vi "DAC Run.vi"(8 "error in":errorcluster, 11 "DAC HS Vib in":refnum<class "DAC HS Vib.lvclass">) -> (0 "error out":errorcluster, 3 "DAC HS Vib out":refnum<class "DAC HS Vib.lvclass">)   [LabVIEW 2019, in "DAC.lvlib" / "DAC HS Vib.lvclass"]
uses:
  DAC HS Vib.lvclass
  C:/Users/krio/Documents/LV_Projects/test-stand/App/DAC/DAC.lvclass
  DAC.lvclass/DAC.ctl
  Results/Results Method.ctl
  Results/DeepU Results/DeepU Results.lvclass
  DAC HS Vib.lvclass/DAC HS Vib.ctl
  <vilib>/DAQmx/read.llb/DAQmx Read (Analog 1D Wfm NChan NSamp).vi
  <vilib>/DAQmx/miscellaneous.llb/DAQmx Fill In Error Info.vi
  DAC.lvclass
  Results/Results.lvlib
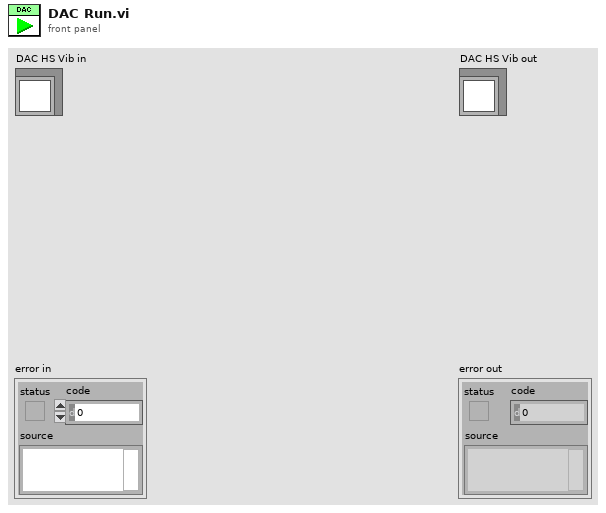
[diagram p1: front panel]
types:
  T1 = typedef "Results.lvlib/Results Method.ctl" = enum16{"Get", "Set"}
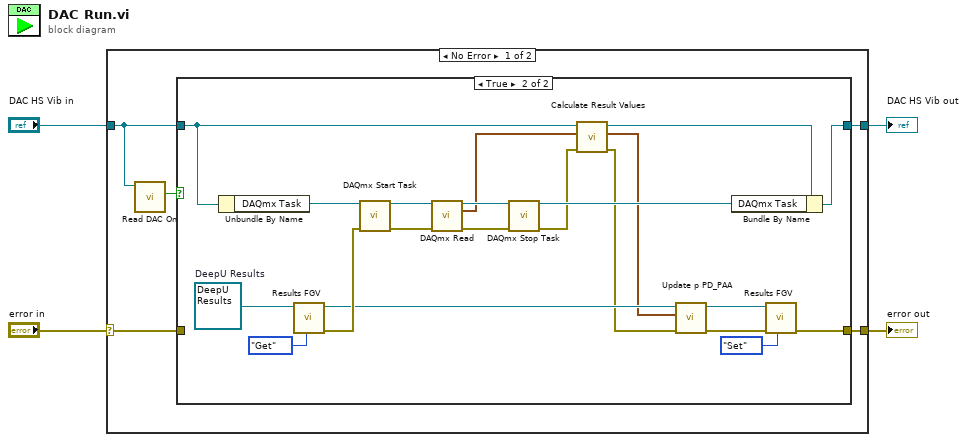
[diagram p0: block diagram]
diagram:
  n1 = case shown="No Error" "error in" {
    selector: "error in" -> [w7 w34]
    tunnel: [w6 w34] -> w2
    tunnel: [w8 w33] -> w1
    tunnel: "DAC HS Vib in" -> [w5 w33]
    frame No Error {
      n2 = call "Read DAC On.vi"("DAC in"=w5) -> ("DAC On"=w9:bool)  [unwired: 8 in, 2 out]
      n3 = case shown="True" w9 {
        tunnel: w5 -> [w11 w17]
        tunnel: [w11 w27] -> w8
        tunnel: w7 -> [w10 _]
        tunnel: [w10 w22] -> w6
        frame False {
        }
        frame True {
          w25 = refnum<class "DeepU Results.lvclass"> refnum  # DeepU Results
          n4 = Unbundle By Name(w17) -> ("DAQmx Task"=w32:refnum<k21>)
          n5 = call-dynamic "Results FGV.vi"("Method"=Results_Method."Get", "DeepU Results in"=w25) -> ("error out"=w21:errorcluster, "DeepU Results out"=w19:refnum<class "DeepU Results.lvclass">)  [unwired: 8 in]
          n6 = call <vilib>:"DAQmx Start Task.vi"("task/channels in"=w32, "error in"=w21) -> ("task out"=w31:refnum<k21>, "error out"=w29:errorcluster)  [unwired: 12 in]
          n7 = call-poly <vilib>:"DAQmx Read.vi"("task/channels in"=w31, "error in"=w29) -> ("task out"=w30:refnum<k21>, "data"=w15:waveform(dbl)[], "error out"=w28:errorcluster)  [unwired: 11 in]
          n8 = call <vilib>:"DAQmx Stop Task.vi"("task/channels in"=w30, "error in"=w28) -> ("task out"=w26:refnum<k21>, "error out"=w14:errorcluster)  [unwired: 12 in]
          n9 = call "Calculate Result Values.vi"("error in"=w14, "Signals in"=w15, "DAC Keller BNC in"=w17) -> ("error out"=w13:errorcluster, "Signals out"=w12:waveform(dbl)[], "DAC Keller BNC out"=w16:refnum<class "DAC HS Vib.lvclass">)  [unwired: 6 in]
          n10 = call "Update p PD_PAA.vi"("error in"=w13, "p PD PAA"=w12, "DeepU Results in"=w19) -> ("error out"=w20:errorcluster, "DeepU Results out"=w18:refnum<class "DeepU Results.lvclass">)  [unwired: 7 in]
          n11 = Bundle By Name(cluster=w16, "DAQmx Task"=w26) -> (w27:refnum<class "DAC HS Vib.lvclass">)
          n12 = call-dynamic "Results FGV.vi"("Method"=Results_Method."Set", "error in"=w20, "DeepU Results in"=w18) -> ("error out"=w22:errorcluster)  [unwired: 7 in, 1 out]
        }
      }
    }
    frame Error {
    }
  }
  "error out" <- w2
  "DAC HS Vib out" <- w1
